vi "ma_resample single-shot (coerce).vi"(6 "#elements":i32, 7 "coerced sample":u16(ring) items=["nearest", "previous", "next"], 8 "error in":errorcluster, 9 "t0":timestamp format="%<%.4X>T", 10 "dt":dbl=1.0 format="%.2p", 11 "waveform in":waveform(dbl)) -> (0 "error out":errorcluster, 3 "resampled waveform out":waveform(dbl))   [LabVIEW 2020, in "NI_MAPro.lvlib"]
doc: "This VI re-samples an unevenly sampled input signal to an evenly sampled waveform according to specified t0 and dt. If the specified t0 value is less than the first value of input X-array (that is the timestamp of the first input sample), then the VI will coerce t0 to the first valid value (greater than X(0)) that also fulfill the relation:\n\nT0_adjusted - t0_in = n * dt_in\n\nThis guarranty that any later comparison of waveforms will be correct with repsect to absolute time."
uses:
  NI_MAPro.lvlib
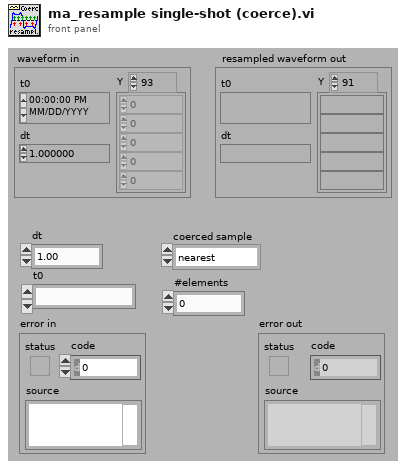
[diagram p1: front panel]
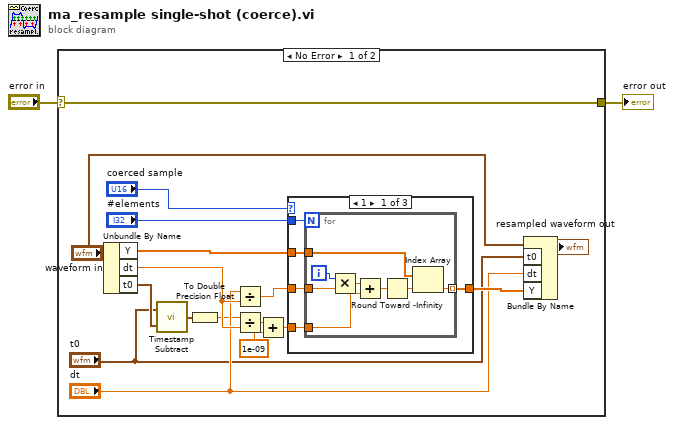
[diagram p0: block diagram]
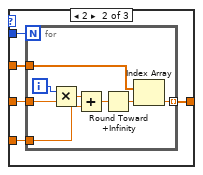
[diagram p2: hidden frame]
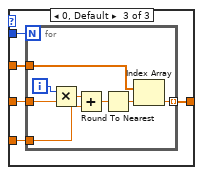
[diagram p3: hidden frame]
diagram:
  n1 = case shown="No Error" "error in" {
    selector: "error in" -> [w7 w59]
    tunnel: [w7 w59] -> w1
    frame No Error {
      n2 = Unbundle By Name("waveform in") -> ("Y"=w17:dbl[], "dt"=w14:dbl, "t0"=w6:timestamp)
      n3 = call "Timestamp Subtract.vi"("y"=w6, "x"="t0") -> ("x - y"=w4:timestamp)
      n4 = To Double Precision Float(number=w4) -> (double precision float=w3:dbl)
      n5 = Divide(x="dt", y=w14) -> (x/y=w15:dbl)
      n6 = Divide(x=w3, y=w14) -> (x/y=w10:dbl)
      n7 = Add(x=w10, y=1e-09) -> (x+y=w8:dbl)
      n8 = case shown="1" "coerced sample" {
        tunnel: "#elements" -> [w24 w37 w50]
        tunnel: w17 -> [w23 w36 w49]
        tunnel: [w22 w35 w48] -> w16
        tunnel: w15 -> [w21 w34 w47]
        tunnel: w8 -> [w20 w33 w46]
        frame 1 {
          n9 = for {
            N: w24 -> [_]
            tunnel: w21 -> [w31]
            tunnel: w23 -> [w28]
            tunnel: [w27] -> w22 mode=indexing
            tunnel: w20 -> [w29]
            i -> [w32]
            n10 = Multiply(x=w32, y=w31) -> (x*y=w30:dbl)
            n11 = Add(x=w30, y=w29) -> (x+y=w26:dbl)
            n12 = Round Toward -Infinity(1:w26) -> (0:w25:dbl)
            n13 = Index Array(array=w28, index=w25) -> (element=w27:dbl)
          }
        }
        frame 2 {
          n14 = for {
            N: w37 -> [_]
            tunnel: w34 -> [w44]
            tunnel: w36 -> [w41]
            tunnel: [w40] -> w35 mode=indexing
            tunnel: w33 -> [w42]
            i -> [w45]
            n15 = Multiply(x=w45, y=w44) -> (x*y=w43:dbl)
            n16 = Add(x=w43, y=w42) -> (x+y=w39:dbl)
            n17 = Round Toward +Infinity(x=w39) -> (ceil(x): smallest int >= x=w38:dbl)
            n18 = Index Array(array=w41, index=w38) -> (element=w40:dbl)
          }
        }
        frame 0, Default {
          n19 = for {
            N: w50 -> [_]
            tunnel: w47 -> [w57]
            tunnel: w49 -> [w54]
            tunnel: [w53] -> w48 mode=indexing
            tunnel: w46 -> [w55]
            i -> [w58]
            n20 = Multiply(x=w58, y=w57) -> (x*y=w56:dbl)
            n21 = Add(x=w56, y=w55) -> (x+y=w52:dbl)
            n22 = Round To Nearest(number=w52) -> (nearest integer value=w51:dbl)
            n23 = Index Array(array=w54, index=w51) -> (element=w53:dbl)
          }
        }
      }
      n24 = Bundle By Name(cluster="waveform in", "t0"="t0", "dt"="dt", "Y"=w16) -> (→"resampled waveform out":waveform(dbl))
    }
    frame Error {
    }
  }
  "error out" <- w1
